vi "test-linear-system-loop-udpate-two-state.vi"(8 "Linearsystem":T1, 9 "Noise":dbl, 10 "dt_Seconds":dbl, 11 "Linear System Loop":T3) -> (1 "CalcYErr":bool, 2 "PredictError":bool, 3 "out Linear System Loop":T3, 4 "CorrectError":bool)   [LabVIEW 2019]
uses:
  <vilib>/Rock Robotics/WPI/ThirdParty/JAS_Junk/TrajLib/LINEAR_SYSTEM_LOOP.ctl
  <vilib>/Rock Robotics/WPI/ThirdParty/JAS_Junk/TrajLib/LINEAR_QUADRATIC_REGULATOR.ctl
  <vilib>/Analysis/Matrix/Datatypes/RealMatrix.ctl
  <vilib>/Rock Robotics/WPI/ThirdParty/JAS_Junk/TrajLib/LINEAR_PLANT_INV_FF.ctl
  <vilib>/Rock Robotics/WPI/ThirdParty/JAS_Junk/TrajLib/KALMAN_FILTER.ctl
  <vilib>/Rock Robotics/WPI/ThirdParty/JAS_Junk/TrajLib/LINEAR_SYSTEM.ctl
  <vilib>/Rock Robotics/WPI/ThirdParty/JAS_Junk/TrajLib/MatBuilder_Create.vi
  <vilib>/Analysis/baseanly.llb/A x B.vi
  <vilib>/Analysis/baseanly.llb/Real A x B.vi
  <vilib>/Rock Robotics/WPI/ThirdParty/JAS_Junk/TrajLib/MatrixHelper_CoerceSize.vi
  <vilib>/Analysis/Matrix/Numeric/Add/Add - RM,RM.vi
  <vilib>/Rock Robotics/WPI/ThirdParty/JAS_Junk/TrajLib/Trajectory_Library.lvlib
  <vilib>/Analysis/Matrix/NI_Matrix.lvlib
panel:
  # "<States,States>"
  # "<States,Inputs>"
  # "<Outputs,States>"
  # "<Outputs,Inputs>"
  # "<States,1>"
  # "<FUTURE --- CLAMP TYPE -- For now\nuse Normalize>"
  # "Steady State Gain  \n<States,Outputs>"
  # "State Estimate <Statess,1>"
  # "<States,States>"
  # "<States,Inputs>"
  # "<Outputs,States>"
  # "<Outputs,Inputs>"
  # "<States,1>"
  # "<Inputs,1>"
  # "<States,Inputs>"
  # "<States,States>"
  # "Ref State <States,1>"
  # "Comp and capped \noutput <Inputs,1>"
  # "Controller gain\n<Inputs,States>"
  # "<States,1>"
  # "<FUTURE --- CLAMP TYPE -- For now\nuse Normalize>"
  # "Steady State Gain  \n<States,Outputs>"
  # "State Estimate <Statess,1>"
  # "<States,States>"
  # "<States,Inputs>"
  # "<Outputs,States>"
  # "<Outputs,Inputs>"
  # "<States,1>"
  # "<Inputs,1>"
  # "<States,Inputs>"
  # "<States,States>"
  # "Ref State <States,1>"
  # "Comp and capped \noutput <Inputs,1>"
  # "Controller gain\n<Inputs,States>"
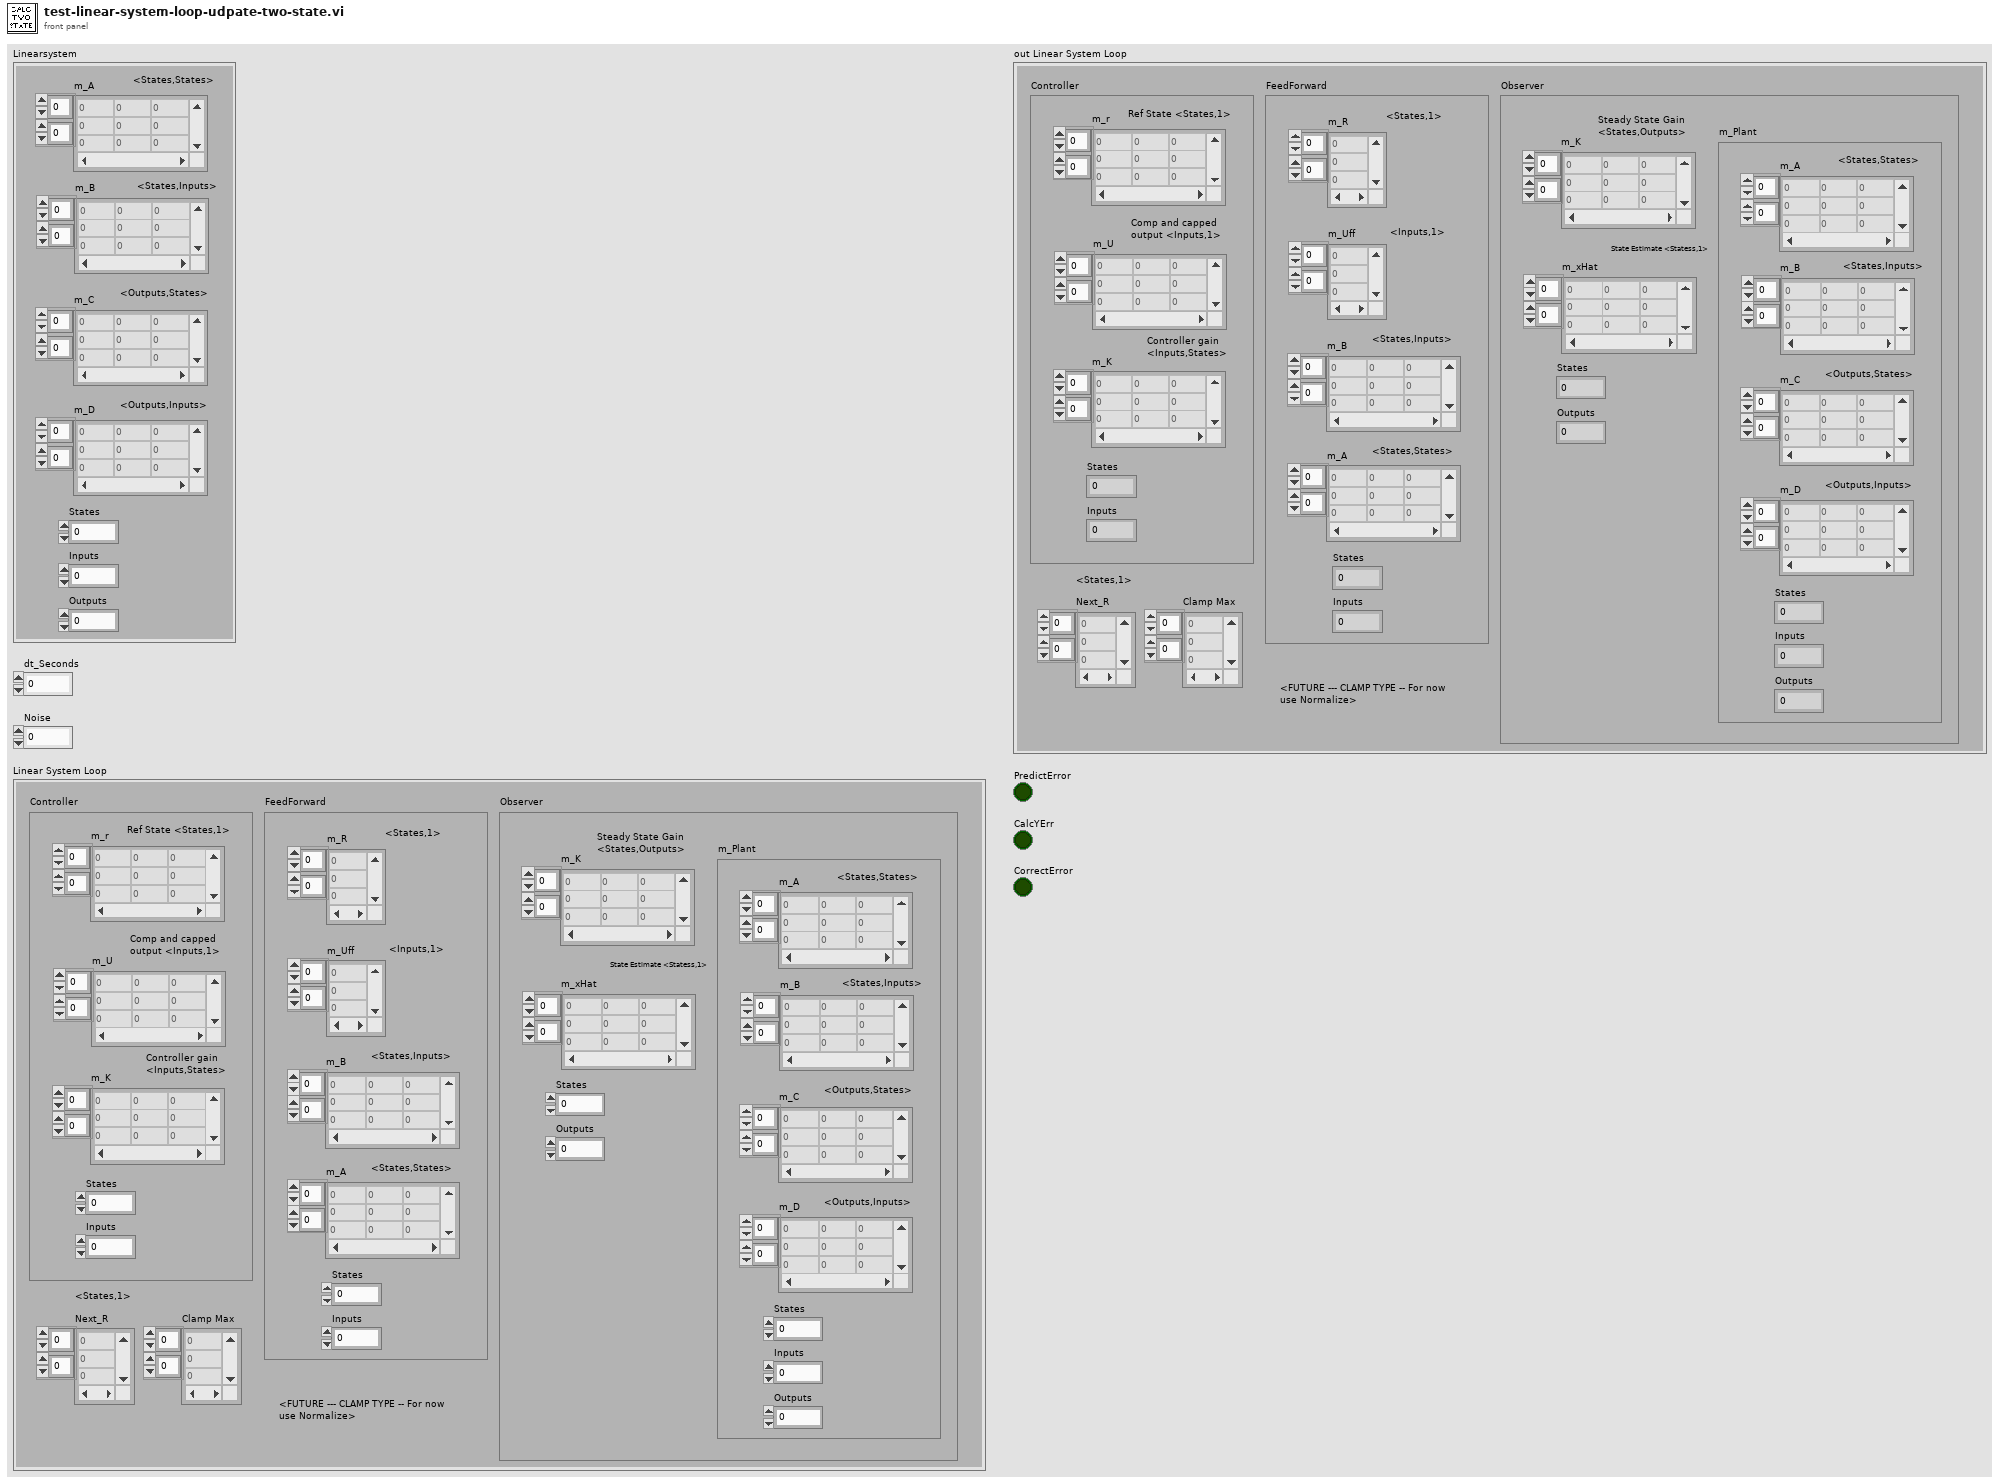
[diagram p1: front panel]
types:
  T1 = typedef "Trajectory_Library.lvlib/LINEAR_SYSTEM.ctl" = cluster{"m_A":T2, "m_B":T2, "m_C":T2, "m_D":T2, "States":i32, "Inputs":i32, "Outputs":i32}
  T2 = typedef "NI_Matrix.lvlib/RealMatrix.ctl" = dbl[][]
  T3 = typedef "Trajectory_Library.lvlib/LINEAR_SYSTEM_LOOP.ctl" = cluster{"Controller":T4, "FeedForward":T5, "Observer":T6, "Next_R":T2, "Clamp Max":T2}
  T4 = typedef "Trajectory_Library.lvlib/LINEAR_QUADRATIC_REGULATOR.ctl" = cluster{"m_r":T2, "m_U":T2, "m_K":T2, "States":i32, "Inputs":i32}
  T5 = typedef "Trajectory_Library.lvlib/LINEAR_PLANT_INV_FF.ctl" = cluster{"m_R":T2, "m_Uff":T2, "m_B":T2, "m_A":T2, "States":i32, "Inputs":i32}
  T6 = typedef "Trajectory_Library.lvlib/KALMAN_FILTER.ctl" = cluster{"m_K":T2, "m_xHat":T2, "States":i32, "Outputs":i32, "m_Plant":T1}
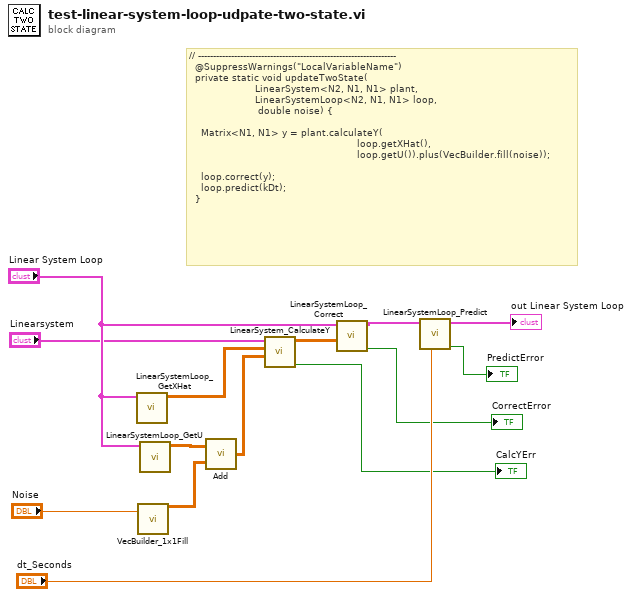
[diagram p0: block diagram]
diagram:
  # "// ------------------------------------------------------------------\n  @SuppressWarnings(\"LocalVariableName\")\n  private static void updateTwoState(\n                      LinearSystem<N2, N1, N1> plant, \n                      LinearSystemLoop<N2, N1, N1> loop, \n                       double noise) {\n\n    Matrix<N1, N1> y = plant.calculateY(\n                                                        loop.getXHat(), \n                                                        loop.getU()).plus(VecBuilder.fill(noise));\n\n    loop.correct(y);\n    loop.predict(kDt);\n  }"
  n1 = call <vilib>:"LinearSystemLoop_GetXHat.vi"("input inear System Loop"="Linear System Loop") -> ("XHat"=w2:T2)  [unwired: 10 in]
  n2 = call <vilib>:"VecBuilder_1x1Fill.vi"("R0_C0"="Noise") -> ("output matrix"=w5:T2)  [unwired: 10 in]
  n3 = call <vilib>:"LinearSystemLoop_GetU.vi"("input inear System Loop"="Linear System Loop") -> ("U"=w4:T2)  [unwired: 10 in]
  n4 = call-poly <vilib>:"Add.vi"("Real Matrix B"=w5, "Real Matrix A"=w4) -> ("A + B"=w6:T2)
  n5 = call <vilib>:"LinearSystem_CalculateY.vi"("ClampedU"=w6, "X"=w2, "Linearsystem"="Linearsystem") -> ("Error"=→"CalcYErr":bool, "outY"=w11:T2)  [unwired: 7 in]
  n6 = call <vilib>:"LinearSystemLoop_Correct.vi"("Y"=w11, "input inear System Loop"="Linear System Loop") -> ("Error"=→"CorrectError":bool, "out Linear System Loop"=w9:T3)  [unwired: 8 in]
  n7 = call <vilib>:"LinearSystemLoop_Predict.vi"("dT_Seconds"="dt_Seconds", "input inear System Loop"=w9) -> ("Error"=→"PredictError":bool, "out Linear System Loop"=→"out Linear System Loop":T3)  [unwired: 8 in]
